vi "GetADCTester (SubVI).vi"(8 "error in (no error)":errorcluster, 9 "GetADCTester":T1(ring), 10 "TimeToGet":i32, 11 "VISA Refnum in":refnum<visa-resource-name>) -> (0 "error out":errorcluster, 2 "ADCValOutput Single":dbl, 3 "ADCValOutput Arr":dbl[](array[numeric]))   [LabVIEW 2017]
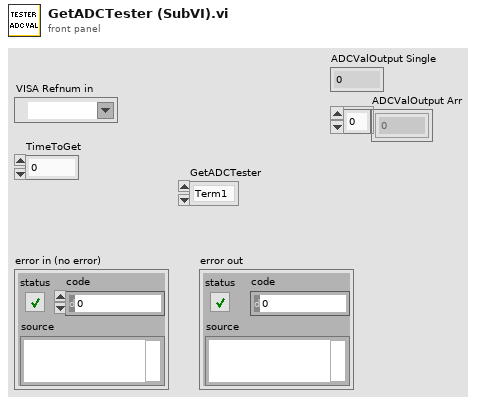
[diagram p1: front panel]
types:
  T1 = enum8{"Term1", "Term2", "Current", "Fan", "TempCPU"}
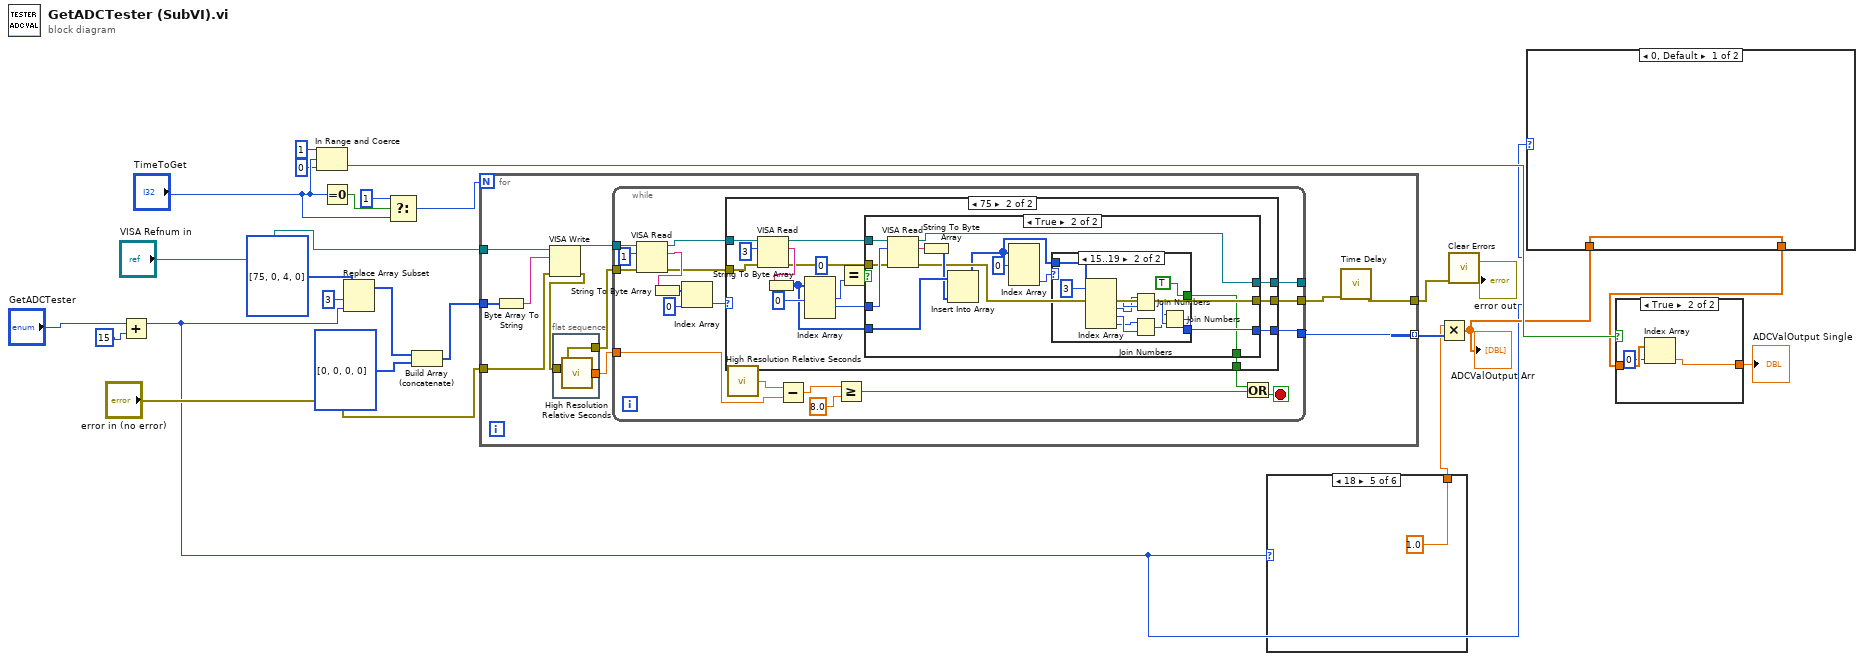
[diagram p0: block diagram]
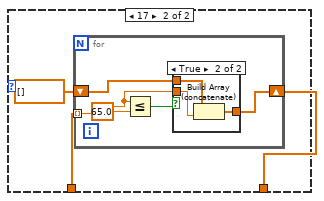
[diagram p2: hidden frame]
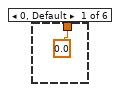
[diagram p4: hidden frame]
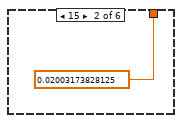
[diagram p5: hidden frame]
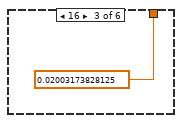
[diagram p6: hidden frame]
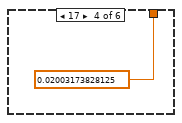
[diagram p7: hidden frame]
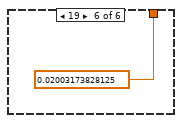
[diagram p8: hidden frame]
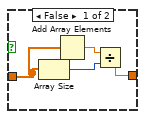
[diagram p9: hidden frame]
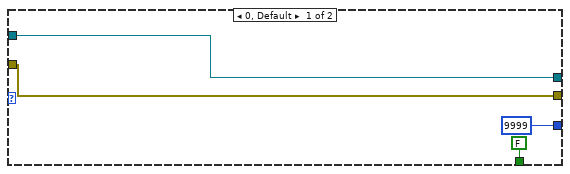
[diagram p10: hidden frame]
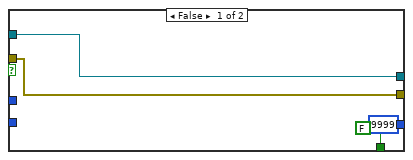
[diagram p11: hidden frame]
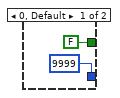
[diagram p12: hidden frame]
diagram:
  n1 = Add(x="GetADCTester", y=u8 15) -> (x+y=w1:u8)
  n2 = In Range and Coerce(upper limit=1, x="TimeToGet", lower limit=0) -> (In Range?=w9:bool)  [unwired: 1 out]
  n3 = Equal To 0?(x="TimeToGet") -> (x = 0?=w22:bool)
  n4 = Replace Array Subset(array=u8[] [75, 0, 4, 0], new element=w1, index=3) -> (w18:u8[])
  n5 = Select(t=1, s=w22, f="TimeToGet") -> (s? t:f=w23:i32)
  n6 = Build Array (concatenate)(w18, u8[] [0, 0, 0, 0]) -> (w19:u8[])
  n7 = for {
    N: w23 -> [_]
    tunnel: "VISA Refnum in" -> [w33]
    tunnel: w19 -> [w32]
    tunnel: [w30] -> w10 mode=indexing
    tunnel: "error in (no error)" -> [w27]
    tunnel: [w25] -> w20
    n8 = Byte Array To String(unsigned byte array=w32) -> (string=w35:string)
    n9 = VISA Write(VISA resource name=w33, write buffer=w35, error in (no error)=w27) -> (VISA resource name out=w34:refnum<visa-resource-name>, error out=w28:errorcluster)  [unwired: 1 out]
    n10 = flat-sequence {
      tunnel: [w37] -> w26
      tunnel: w28 -> [w36]
      tunnel: [w36] -> w29
      frame #0 {
        n11 = call <vilib>:"High Resolution Relative Seconds.vi"() -> ("relative seconds"=w37:dbl)
      }
    }
    n12 = while {
      tunnel: w34 -> [w49]
      tunnel: w29 -> [w48]
      tunnel: [w47] -> _
      tunnel: [w46] -> w31
      tunnel: [w45] -> w30
      tunnel: w26 -> [w42]
      stop <- w44 stop-if-true
      n13 = VISA Read(VISA resource name=w49, byte count=u32 1, error in (no error)=w48) -> (VISA resource name out=w51:refnum<visa-resource-name>, read buffer=w52:string, error out=w50:errorcluster)  [unwired: 1 out]
      n14 = String To Byte Array(string=w52) -> (unsigned byte array=w55:u8[])
      n15 = Index Array(array=w55, index=0) -> (element=w53:u8)
      n16 = case shown="75" w53 {
        tunnel: [w60 w64] -> w46
        tunnel: w51 -> [w59 w73]
        tunnel: w50 -> [w60 w72]
        tunnel: [w59 w65] -> w47
        tunnel: [u32 9999 w62] -> w45
        tunnel: [FALSE w61] -> w43
        frame 0, Default {
        }
        frame 75 {
          n17 = VISA Read(VISA resource name=w73, byte count=u32 3, error in (no error)=w72) -> (VISA resource name out=w68:refnum<visa-resource-name>, read buffer=w76:string, error out=w67:errorcluster)  [unwired: 1 out]
          n18 = String To Byte Array(string=w76) -> (unsigned byte array=w66:u8[])
          n19 = Index Array(array=w66, index #1=0 ("index")) -> (element #1=w71:u8, element #2=w69:u8)  [unwired: 2 in, 1 out]
          n20 = Equal?(x=u8 0, y=w71) -> (x = y?=w70:bool)
          n21 = case shown="True" w70 {
            tunnel: [w79 w86] -> w64
            tunnel: w69 -> [_ w93]
            tunnel: w68 -> [w80 w92]
            tunnel: w67 -> [w79 w91]
            tunnel: w66 -> [_ w90]
            tunnel: [w80 w88] -> w65
            tunnel: [u32 9999 w82] -> w62
            tunnel: [FALSE w81] -> w61
            frame False {
            }
            frame True {
              n22 = VISA Read(VISA resource name=w92, byte count=w93, error in (no error)=w91) -> (VISA resource name out=w88:refnum<visa-resource-name>, read buffer=w87:string, error out=w86:errorcluster)  [unwired: 1 out]
              n23 = String To Byte Array(string=w87) -> (unsigned byte array=w89:u8[])
              n24 = Insert Into Array(array=w90, new element=w89) -> (w83:u8[])  [unwired: 1 in]
              n25 = Index Array(array=w83, index #1=0 ("index")) -> (element #3=w84:u8)  [unwired: 2 in, 2 out]
              n26 = case shown="15..19" w84 {
                tunnel: w83 -> [_ w104]
                tunnel: [u32 9999 w97] -> w82
                tunnel: [FALSE TRUE] -> w81
                frame 0, Default {
                }
                frame 15..19 {
                  n27 = Index Array(array=w104, index #1=3 ("index")) -> (element #1=w103:u8, element #2=w102:u8, element #3=w101:u8, element #4=w100:u8)  [unwired: 3 in]
                  n28 = Join Numbers(hi=w102, lo=w103) -> ((hi.lo)=w99:u16)
                  n29 = Join Numbers(hi=w100, lo=w101) -> ((hi.lo)=w98:u16)
                  n30 = Join Numbers(hi=w98, lo=w99) -> ((hi.lo)=w97:u32)
                }
              }
            }
          }
        }
      }
      n31 = call <vilib>:"High Resolution Relative Seconds.vi"() -> ("relative seconds"=w41:dbl)
      n32 = Subtract(x=w41, y=w42) -> (x-y=w40:dbl)
      n33 = Greater Or Equal?(x=w40, y=8.0) -> (x >= y?=w38:bool)
      n34 = Or(x=w43, y=w38) -> (x .or. y?=w44:bool)
    }
    n35 = call "Time Delay"("error in (no error)"=w31) -> ("error out"=w25:errorcluster)  [unwired: 10 in]
  }
  n36 = case shown="18" w1 {
    tunnel: [0.0 ("x") 0.02003173828125 ("x") 0.02003173828125 ("x") 0.02003173828125 ("x") 1.0 ("x") 0.02003173828125 ("x")] -> w4
    frame 0, Default {
    }
    frame 15 {
    }
    frame 16 {
    }
    frame 17 {
    }
    frame 18 {
    }
    frame 19 {
    }
  }
  n37 = Multiply(x=w4, y=w10) -> (x*y=w3:dbl[])
  "ADCValOutput Arr" <- w3
  n38 = call <vilib>:"Clear Errors.vi"("error in (no error)"=w20) -> ("error out"=→"error out":errorcluster)  [unwired: 5 in, 1 out]
  n39 = case shown="0, Default" w1 {
    tunnel: w3 -> [w112 w115]
    tunnel: [w112 w113] -> w2
    frame 0, Default {
    }
    frame 17 {
      n40 = for {
        tunnel: w115 -> [w118] mode=indexing
        shift-right: [w116] -> w113
        shift-left: dbl[] [] -> [w117]
        n41 = Less Or Equal?(x=w118, y=65.0) -> (x <= y?=w119:bool)
        n42 = case shown="True" w119 {
          tunnel: w118 -> [_ w124]
          tunnel: [w121 w123] -> w116
          tunnel: w117 -> [w121 w122]
          frame False {
          }
          frame True {
            n43 = Build Array (concatenate)(w122, w124) -> (w123:dbl[])
          }
        }
      }
    }
  }
  n44 = case shown="True" w9 {
    tunnel: w2 -> [w128 w131]
    tunnel: [w125 w129] -> w8
    frame False {
      n45 = Array Size(array=w128) -> (size(s)=w126:i32)
      n46 = Add Array Elements(numeric array=w128) -> (sum=w127:dbl)
      n47 = Divide(x=w127, y=w126) -> (x/y=w125:dbl)
    }
    frame True {
      n48 = Index Array(array=w131, index=0) -> (element=w129:dbl)
    }
  }
  "ADCValOutput Single" <- w8
